vi "PH_DataViewer.allocate or free img space.vi"(0 "i ref in":refnum<vi>, 2 "Allocate?":bool, 5 "error in (no error)":errorcluster) -> (14 "i ref out":refnum<vi>, 19 "error out":errorcluster)   [LabVIEW 2014, in "PH_DataViewer.lvlib"]
doc: "This VI is forseen to be used in constructor or destructor. If Allocate? = true is chosen, memory space for several images is allocated. If false is chosen, it is freed."
uses:
  PH_DataViewer.lvlib
  CS_Core/CSSystem/CSSystemLib/CSSystemLib.lvlib
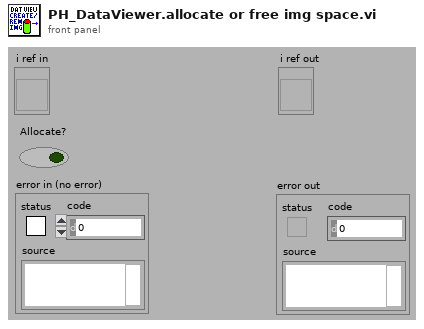
[diagram p1: front panel]
types:
  T1 = typedef "PH_DataViewer.lvlib/PH_DataViewer.i attribute.ctl" = cluster{"Images":cluster{"CAM":cluster{string, u32}, "BACKGROUND":cluster{string, u32}, "OPERATOR":cluster{string, u32}}, "Cam Operator GUI Refs":cluster{"Date Operators":refnum<vi>, "Time Operators":refnum<vi>, "Status Cali Data":refnum<vi>, "Calibration data":refnum<vi>, "Background Image":refnum<vi>, "Bg subtracted":refnum<vi>, "Op Image":refnum<vi>, "Cam Settings Operator":refnum<vi>, "Energy on":refnum<vi>, "exp Energy":refnum<vi>, "Energy":refnum<vi>, "Beam Analysis":refnum<vi>, "Analysis Type":refnum<vi>, "BA: Steps":refnum<vi>, "BA: Factor for ROI":refnum<vi>, "CoG - X":refnum<vi>, "CoG - Y":refnum<vi>, "Maj Diam":refnum<vi>, "Min Diam":refnum<vi>, "Phi":refnum<vi>, "Epsilon":refnum<vi>, "Phi rel to maj":refnum<vi>, "Position":refnum<vi>, "Position Type":refnum<vi>, "exp - X":refnum<vi>, "exp - Y":refnum<vi>, "Magni":refnum<vi>, "Foc Length":refnum<vi>, "Delta":refnum<vi>, "Theta":refnum<vi>, "Fit Gauss":refnum<vi>, "Maj Fit Order":refnum<vi>, "Min Fit Order":refnum<vi>, "Maj FWHM":refnum<vi>, "Min FWHM":refnum<vi>, "Maj 1 %":refnum<vi>, "Min 1 %":refnum<vi>}}
  T2 = cluster{"CAM":cluster{string, u32}, "BACKGROUND":cluster{string, u32}, "OPERATOR":cluster{string, u32}}
  T3 = typedef "IMAQ Image.ctl" = refnum<image>
  T4 = typedef "Image Type" = u32
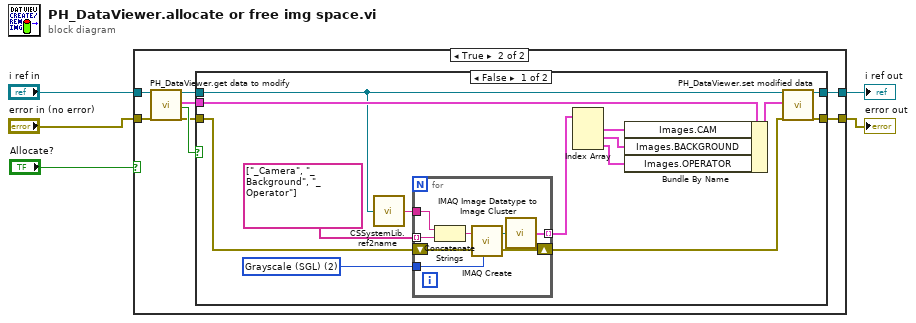
[diagram p0: block diagram]
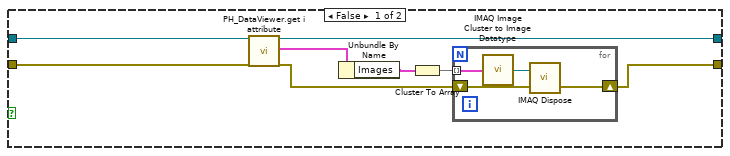
[diagram p2: hidden frame]
diagram:
  n1 = case shown="True" "Allocate?" {
    tunnel: [w8 w24] -> w5
    tunnel: [w10 w23] -> w4
    tunnel: "error in (no error)" -> [w13 w20]
    tunnel: "i ref in" -> [w12 w19]
    frame False {
      n2 = call "PH_DataViewer.get i attribute.vi"("i ref in"=w12, "error in (no error)"=w13) -> ("i ref out"=w10:refnum<vi>, "i attribute"=w11:T1, "error out"=w9:errorcluster)  [unwired: 15 in]
      n3 = Unbundle By Name(w11) -> ("Images"=w7:T2)
      n4 = Cluster To Array(cluster=w7) -> (array=w6:cluster{string, u32}[])
      n5 = for {
        shift-right: [w16] -> w8
        shift-left: w9 -> [w17]
        tunnel: w6 -> [w15] mode=indexing
        n6 = call <vilib>:"IMAQ Image Cluster to Image Datatype.vi"("Image"=w15) -> ("Image (dup)"=w14:T3)
        n7 = call "IMAQ Dispose"("Image"=w14, "error in (no error)"=w17) -> ("error out"=w16:errorcluster)  [unwired: 4 in]
      }
    }
    frame True {
      n8 = call "PH_DataViewer.get data to modify.vi"("i ref in"=w19, "error in (no error)"=w20) -> ("i ref out"=w22:refnum<vi>, "i attribute"=w18:T1, "timed out"=w25:bool, "error out"=w21:errorcluster)  [unwired: 14 in]
      n9 = case shown="False" w25 {
        tunnel: w21 -> [w34 w48]
        tunnel: w22 -> [w27 w49]
        tunnel: [w39 w49] -> w23
        tunnel: [w38 w48] -> w24
        tunnel: w18 -> [w37 _]
        frame False {
          w29 = T4 2 items=["Grayscale (U8)", "Grayscale (I16)", "Grayscale (SGL)", "Complex (CSG)", "RGB (U32)", "HSL (U32)", "RGB (U64)"] ("Image Type")
          n10 = call "CSSystemLib.ref2name.vi"("obj refnum"=w27) -> ("name"=w26:string)
          n11 = for {
            shift-right: [w47] -> w35
            shift-left: w34 -> [w46]
            tunnel: [w43] -> w33 mode=indexing
            tunnel: string[] ["_Camera", "_Background", "_Operator"] -> [w41] mode=indexing
            tunnel: w29 -> [w45]
            tunnel: w26 -> [w42]
            n12 = Concatenate Strings(w42, w41) -> (w40:string)
            n13 = call "IMAQ Create"("Image Name"=w40, "Image Type"=w45, "error in (no error)"=w46) -> ("New Image"=w44:T3, "error out"=w47:errorcluster)  [unwired: 2 in]
            n14 = call <vilib>:"IMAQ Image Datatype to Image Cluster.vi"("Image"=w44) -> ("Image (dup)"=w43:cluster{string, u32})
          }
          n15 = Index Array(array=w33) -> (element #1=w31:cluster{string, u32}, element #2=w30:cluster{string, u32}, element #3=w28:cluster{string, u32})  [unwired: 3 in]
          n16 = Bundle By Name(cluster=w37, "Images.CAM"=w31, "Images.BACKGROUND"=w30, "Images.OPERATOR"=w28) -> (w36:T1)
          n17 = call "PH_DataViewer.set modified data.vi"("i ref in"=w27, "i attribute"=w36, "error in (no error)"=w35) -> ("i ref out"=w39:refnum<vi>, "error out"=w38:errorcluster)  [unwired: 15 in]
        }
        frame True {
        }
      }
    }
  }
  "error out" <- w5
  "i ref out" <- w4
